vi "CB Serial Test_v2.vi"(8 "error in (no error)":errorcluster, 11 "ControlBoard VISA":refnum<visa-resource-name>="ControlBoard") -> (0 "error out":errorcluster, 2 "Actual Result":string, 3 "Pass/Fail":bool)   [LabVIEW 2022 SP3]
doc: "This VI will compare the serial menu printed by an EPC blue board to a reference and determine a pass or fail"
uses:
  <vilib>/Instr/_visa.llb/VISA Flush IO Buffer Mask.ctl
panel:
  out "Expected Result":string
  out "VISA resource OUT":refnum<visa-resource-name>
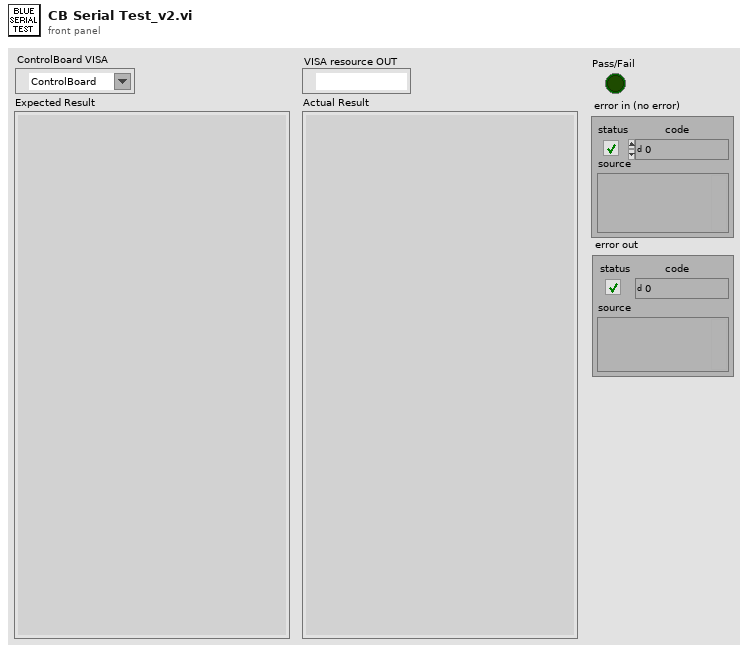
[diagram p1: front panel]
types:
  T1 = typedef "VISA Flush IO Buffer Mask.ctl" = u16
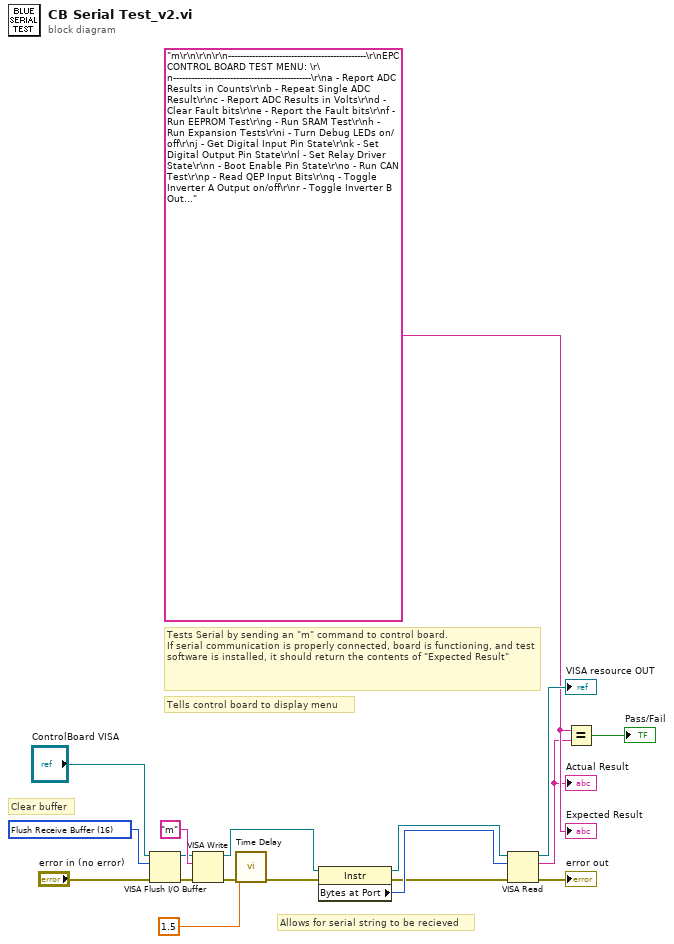
[diagram p0: block diagram]
diagram:
  w6 = "m\r\n\r\n\r\n----------------------------------------------\r\nEPC CONTROL BOARD TEST MENU: \r\n----------------------------------------------\r\na - Report ADC Results in Counts\r\nb - Repeat Single ADC Result\r\nc - Report ADC Results in Volts\r\nd - Clear Fault bits\r\ne - Report the Fault bits\r\nf - Run EEPROM Test\r\ng - Run SRAM Test\r\nh - Run Expansion Tests\r\ni - Turn Debug LEDs on/off\r\nj - Get Digital Input Pin State\r\nk - Set Digital Output Pin State\r\nl - Set Relay Driver State\r\nn - Boot Enable Pin State\r\no - Run CAN Test\r\np - Read QEP Input Bits\r\nq - Toggle Inverter A Output on/off\r\nr - Toggle Inverter B Output on/off\r\ns - Toggle Half Bridge Output on/off\r\nt - Set PWM leg duty cycle\r\nu - Real Time Clock\r\nv - Watchdog Control\r\nw - Test Interrupt Lines\r\nx - Read HALLs\r\ny - Test FPGA Read/Write\r\nz - Report Software/FPGA Revs\r\nm - Display this menu\r\n0 - Report Internal RAM Zeroed\r\n1 - Report SRAM Zeroed\r\n2 - Report SRAM Initialized\r\n3 - Run Quick EEPROM Test\r\n4 - Report Temperature and Humidity\r\n> "
  w15 = T1 16 items=["Flush Receive Buffer"=16, "Write Transmit Buffer to Device"=32, "Flush Receive Buffer (No I/O)"=64, "Flush Transmit Buffer"=128] ("Mask")
  # "Tests Serial by sending an \"m\" command to control board.\nIf serial communication is properly connected, board is functioning, and test software is installed, it should return the contents of \"Expected Result\""
  # "Clear buffer"
  # "Allows for serial string to be recieved"
  # "Tells control board to display menu"
  n1 = VISA Flush I/O Buffer(VISA resource name="ControlBoard VISA", mask (16)=w15, error in (no error)="error in (no error)") -> (VISA resource name out=w13:refnum<visa-resource-name>, error out=w12:errorcluster)
  n2 = VISA Write(VISA resource name=w13, write buffer="m", error in (no error)=w12) -> (VISA resource name out=w10:refnum<visa-resource-name>, error out=w14:errorcluster)  [unwired: 1 out]
  n3 = call "Time Delay"("error in (no error)"=w14, "Delay Time (s)"=1.5) -> ("error out"=w11:errorcluster)  [unwired: 9 in]
  n4 = property class="Instr"(reference=w10, error in=w11) -> (reference out=w17:refnum<visa-resource-name>, error out=w3:errorcluster, "Bytes at Port"=w16:u32)
  n5 = VISA Read(VISA resource name=w17, byte count=w16, error in (no error)=w3) -> (VISA resource name out=→"VISA resource OUT":refnum<visa-resource-name>, read buffer=w5:string, error out=→"error out":errorcluster)  [unwired: 1 out]
  "Actual Result" <- w5
  n6 = Equal?(x=w6, y=w5) -> (x = y?=→"Pass/Fail":bool)
  "Expected Result" <- w6
